vi "Extract side Number.vi"() -> ()   [LabVIEW 2015]
uses:
  <vilib>/Utility/file.llb/Read Delimited Spreadsheet (string).vi
  <vilib>/Utility/file.llb/Write Delimited Spreadsheet (string).vi
panel:
  out "filenames":string[](array[string])
  out "String":string
  in  "file path (dialog if empty)":path=path "J:/Sort/TV/path.txt"
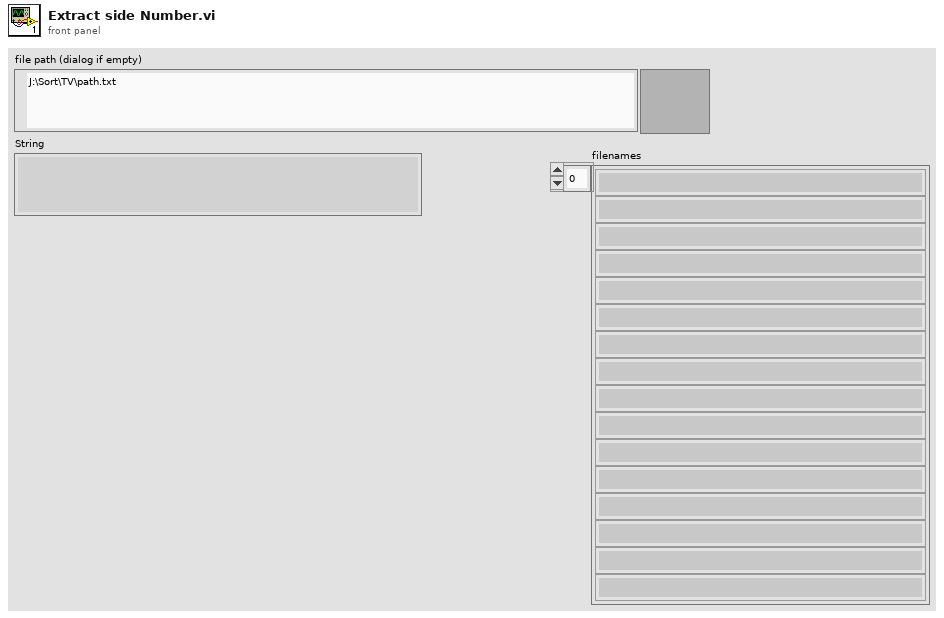
[diagram p1: front panel]
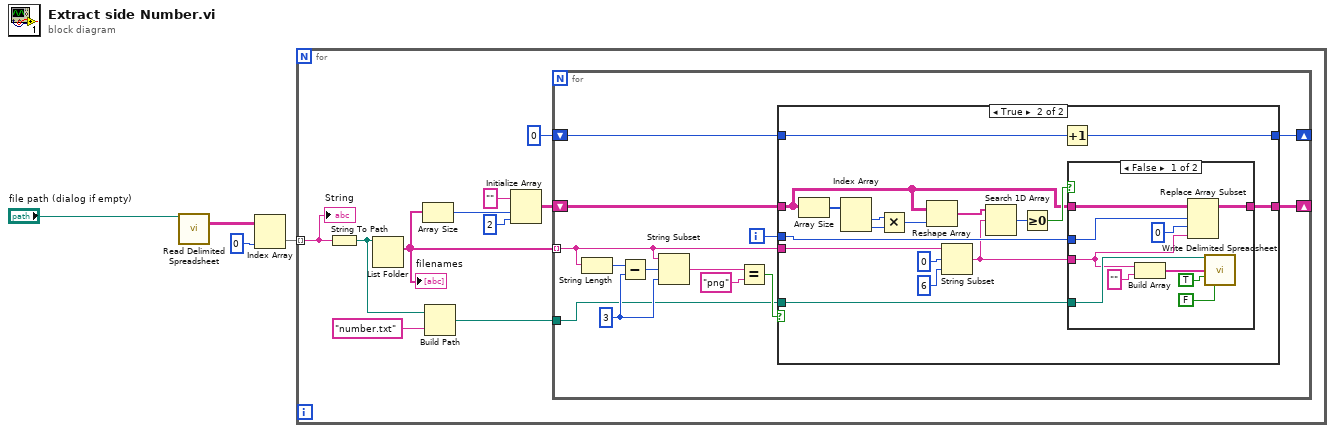
[diagram p0: block diagram]
diagram:
  n1 = call-poly <vilib>:"Read Delimited Spreadsheet.vi"("file path (dialog if empty)"="file path (dialog if empty)") -> ("all rows"=w3:string[][])  [unwired: 9 in, 5 out]
  n2 = Index Array(array=w3, index (col)=0 ("disabled index (col)")) -> (element=w1:string[])  [unwired: 1 in]
  n3 = for {
    tunnel: w1 -> [w14] mode=indexing
    n4 = String To Path(string=w14) -> (path=w13:path)
    n5 = List Folder(path=w13) -> (filenames=w11:string[])  [unwired: 3 in, 3 out]
    "filenames" <- w11
    n6 = Array Size(array=w11) -> (size(s)=w9:i32)
    n7 = Build Path(base path=w13, name or relative path="number.txt") -> (appended path=w5:path)
    n8 = Initialize Array("", w9, 2 ("dimension size")) -> (w7:string[][])
    n9 = for {
      tunnel: w11 -> [w19] mode=indexing
      shift-right: [w18] -> _
      shift-left: w7 -> [w21]
      shift-right: [w16] -> _
      shift-left: 0 ("offset (0)") -> [w17]
      tunnel: w5 -> [w15]
      i -> [w20]
      w25 = 3 ("y")
      n10 = String Length(string=w19) -> (length=w27:i32)
      n11 = Subtract(x=w27, y=w25) -> (x-y=w26:i32)
      n12 = String Subset(string=w19, offset (0)=w26, length (rest)=w25) -> (substring=w24:string)
      n13 = Equal?(x=w24, y="png") -> (x = y?=w22:bool)
      n14 = case shown="True" w22 {
        tunnel: w21 -> [w29 w36]
        tunnel: w20 -> [_ w39]
        tunnel: w19 -> [_ w45]
        tunnel: [w29 w37] -> w18
        tunnel: w17 -> [w28 w44]
        tunnel: [w28 w43] -> w16
        tunnel: w15 -> [_ w30]
        frame False {
        }
        frame True {
          n15 = Array Size(array=w36) -> (size(s)=w35:i32[])
          n16 = Index Array(array=w35) -> (element #1=w34:i32, element #2=w33:i32)  [unwired: 2 in]
          n17 = Multiply(x=w34, y=w33) -> (x*y=w32:i32)
          n18 = Reshape Array(w36, w32) -> (w42:string[])
          n19 = String Subset(string=w45, offset (0)=0, length (rest)=6 ("y")) -> (substring=w38:string)
          n20 = Search 1D Array(1D array=w42, element=w38) -> (index of element=w41:i32)  [unwired: 1 in]
          n21 = Greater Or Equal To 0?(x=w41) -> (x >= 0?=w40:bool)
          n22 = Increment(x=w44) -> (x+1=w43:i32)
          n23 = case shown="False" w40 {
            tunnel: w36 -> [w55 w57]
            tunnel: [w53 w57] -> w37
            tunnel: w39 -> [w54 _]
            tunnel: w38 -> [w51 _]
            tunnel: w30 -> [w52 _]
            frame False {
              n24 = Build Array(w51, "" ("element")) -> (w49:string[])
              n25 = Replace Array Subset(array=w55, new element=w51, index (row)=w54, index (col)=0 ("disabled index (col)")) -> (w53:string[][])
              n26 = call-poly <vilib>:"Write Delimited Spreadsheet.vi"("file path (dialog if empty)"=w52, "1D data"=w49, "append to file? (F)"=TRUE, "transpose? (F)"=FALSE) -> ()  [unwired: 10 in, 2 out]
            }
            frame True {
            }
          }
        }
      }
    }
    "String" <- w14
  }
